vi "Handle Endianity.vi"(8 "error in (no error)":errorcluster, 10 "Bytes to read in":string, 11 "Kasli Listener in":refnum<class "Kasli Listener.lvclass">) -> (0 "error out":errorcluster, 2 "Bytes to read out":string, 3 "Kasli Listener out":refnum<class "Kasli Listener.lvclass">)   [LabVIEW 2020, in "Kasli Listener and Writer.lvlib" / "Kasli Listener.lvclass"]
uses:
  Kasli Listener.lvclass
  Kasli Listener.lvclass/Kasli Listener.ctl
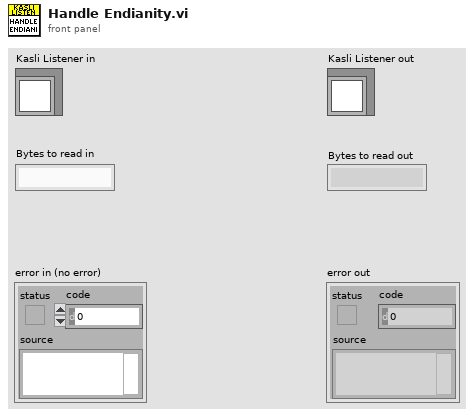
[diagram p1: front panel]
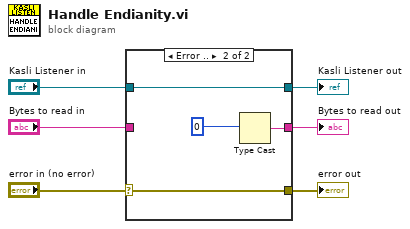
[diagram p0: block diagram]
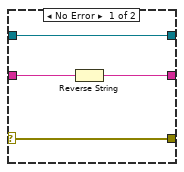
[diagram p2: hidden frame]
diagram:
  n1 = case shown="Error .." "error in (no error)" {
    selector: "error in (no error)" -> [w9 w13]
    tunnel: "Kasli Listener in" -> [w10 w14]
    tunnel: [w10 w14] -> w5
    tunnel: [w9 w13] -> w3
    tunnel: "Bytes to read in" -> [w8 _]
    tunnel: [w7 w11] -> w1
    frame No Error {
      n2 = Reverse String(1:w8) -> (0:w7:string)
    }
    frame Error {
      n3 = Type Cast(x=0) -> (*(type *) &x=w11:string)  [unwired: 1 in]
    }
  }
  "error out" <- w3
  "Kasli Listener out" <- w5
  "Bytes to read out" <- w1
